vi "Tosca-Save AI Layout.vi"(0 "VI in":refnum<vi>, 5 "GraphSplitter":refnum<vi>, 7 "More":bool, 11 "error in (no error)":errorcluster) -> (15 "error out":errorcluster)   [LabVIEW 2020]
uses:
  <vilib>/Utility/miscctls.llb/LVRectTypeDef.ctl
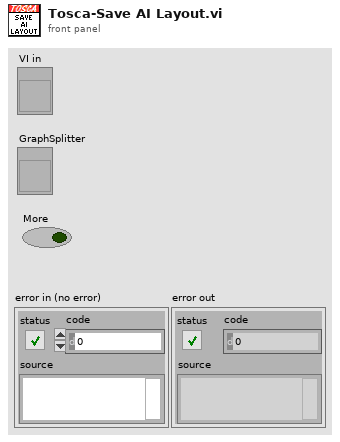
[diagram p1: front panel]
types:
  T1 = typedef "LVRectTypeDef.ctl" = cluster{"Left":i16, "Top":i16, "Right":i16, "Bottom":i16}
  T2 = cluster{"bounds":T1, "splitter":i32, "more":bool}
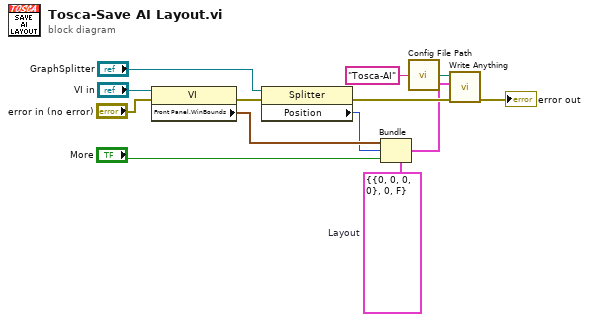
[diagram p0: block diagram]
diagram:
  w5 = T2 {"bounds"={"Left"=0, "Top"=0, "Right"=0, "Bottom"=0}, "splitter"=0, "more"=FALSE}  # Layout
  n1 = property class="VI"(reference="VI in", error in="error in (no error)") -> (error out=w11:errorcluster, "Front Panel.WinBounds"=w9:T1)  [unwired: 1 out]
  n2 = property class="Splitter"(reference="GraphSplitter", error in=w11) -> (error out=w6:errorcluster, "Position"=w8:i32)  [unwired: 1 out]
  n3 = Bundle(cluster=w5, "bounds"=w9, "splitter"=w8, "more"="More") -> (w4:T2)
  n4 = call "Config File Path.vi"("AppName"="Tosca-AI") -> ("Default config file name"=w3:path)
  n5 = call "Write Anything.vi"("Error In"=w6, "Anything"=w4, "Path (dialog)"=w3) -> ("Error Out"=→"error out":errorcluster)  [unwired: 7 in, 1 out]
